vi "Get I32.vi"(8 "error in (no error)":errorcluster, 10 "Name":string, 11 "json class in":refnum<class "json class.lvclass">) -> (0 "error out":errorcluster, 2 "I32":i32, 3 "json class out":refnum<class "json class.lvclass">)   [LabVIEW 2021, in "Config Library.lvlib" / "json class.lvclass"]
uses:
  json class.lvclass
  json class.lvclass/json class.ctl
  <vilib>/addons/JSON API/JSON Scalar/JSON Scalar.lvclass
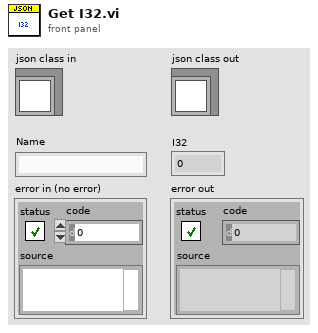
[diagram p1: front panel]
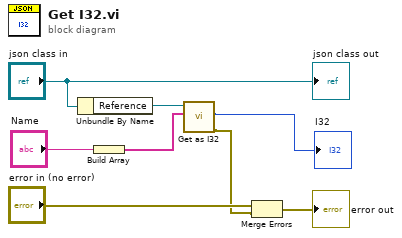
[diagram p0: block diagram]
diagram:
  n1 = Unbundle By Name("json class in") -> ("Reference"=w4:refnum<class "JSON Value.lvclass">)
  n2 = Build Array("Name") -> (w3:string[])
  n3 = call <vilib>:"Get as I32.vi"("Name Array"=w3, "JSON Scalar in"=w4) -> ("error out"=w1:errorcluster, "Number"=→"I32":i32)  [unwired: 7 in, 1 out]
  n4 = Merge Errors("error in (no error)", w1) -> (→"error out":errorcluster)
  "json class out" <- "json class in"
